vi "xeva-getTemperatureSP.vi"(2 "error in (no error)":errorcluster, 3 "xeva-camref":T1) -> (0 "error out":errorcluster, 1 "xeva-temperature-setpoint":dbl)   [LabVIEW 2015]
uses:
  <vilib>/Xenics Infrared Solutions/Xeneth LabVIEW API/VIs/Controls/Camara.ctl
  <vilib>/Xenics Infrared Solutions/Xeneth LabVIEW API/Xeneth.lvlib
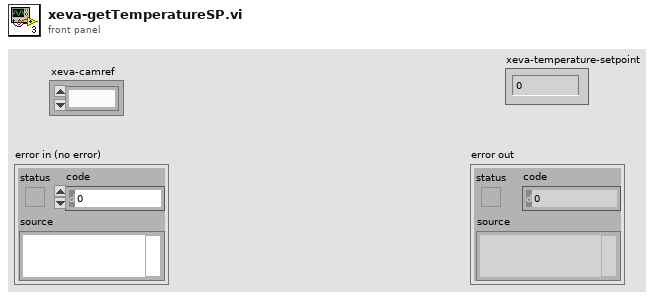
[diagram p1: front panel]
types:
  T1 = typedef "Xeneth.lvlib/Camara.ctl" = refnum<k1>
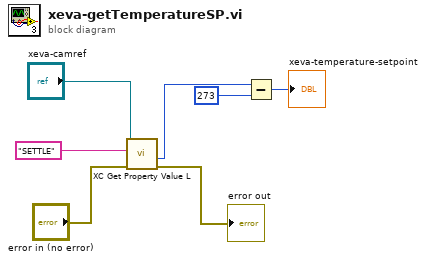
[diagram p0: block diagram]
diagram:
  n1 = call <vilib>:"XC Get Property Value L.vi"("error in (no error)"="error in (no error)", "pPrp"="SETTLE", "Cam Ref"="xeva-camref") -> ("error out"=→"error out":errorcluster, "pValue out"=w3:i32)  [unwired: 6 in, 1 out]
  n2 = Subtract(x=w3, y=273) -> (x-y=→"xeva-temperature-setpoint":i32)
